vi "Calculate_(101)_Global_Cost_F()-1.vi"(5 "[IN] Still connect\ned tracks in group":T1, 6 "[IN] Max angle":dbl, 7 "[IN] Subtracks":T2(array[cluster]), 8 "error IN":errorcluster, 9 "[IN] Areas particles\nPrimary Detected":dbl[][](array[numeric]), 10 "[IN] Primary \n(X,Y) Detected":dbl[][](array[numeric]), 11 "[IN] Cost function":i8[](array[numeric])) -> (0 "error OUT":errorcluster, 3 "[OUT] Cost function":i8[](array[numeric]))   [LabVIEW 2013]
uses:
  <vilib>/Analysis/NI_AALBase.lvlib
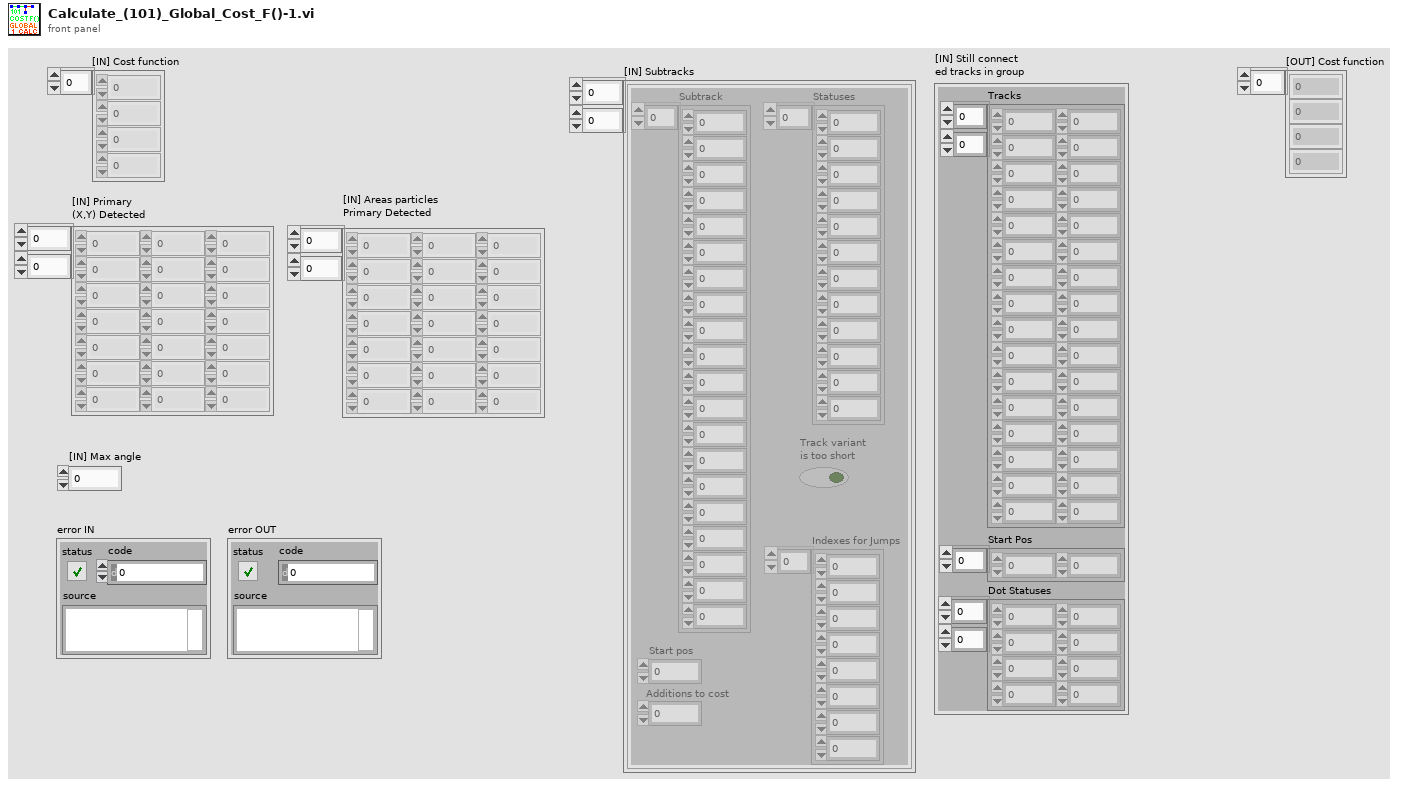
[diagram p1: front panel]
types:
  T1 = cluster{"Tracks":dbl[][], "Start Pos":i32[], "Dot Statuses":i16[][]}
  T2 = cluster{"Subtrack":dbl[], "Statuses":i16[], "Start pos":i32, "Additions to cost":i32, "Track variant \nis too short":bool, "Indexes for Jumps":i32[]}[][]
  T3 = cluster{"Subtrack":dbl[], "Statuses":i16[], "Start pos":i32, "Additions to cost":i32, "Track variant \nis too short":bool, "Indexes for Jumps":i32[]}[]
  T4 = cluster{"Subtrack":dbl[], "Statuses":i16[], "Start pos":i32, "Additions to cost":i32, "Track variant \nis too short":bool, "Indexes for Jumps":i32[]}
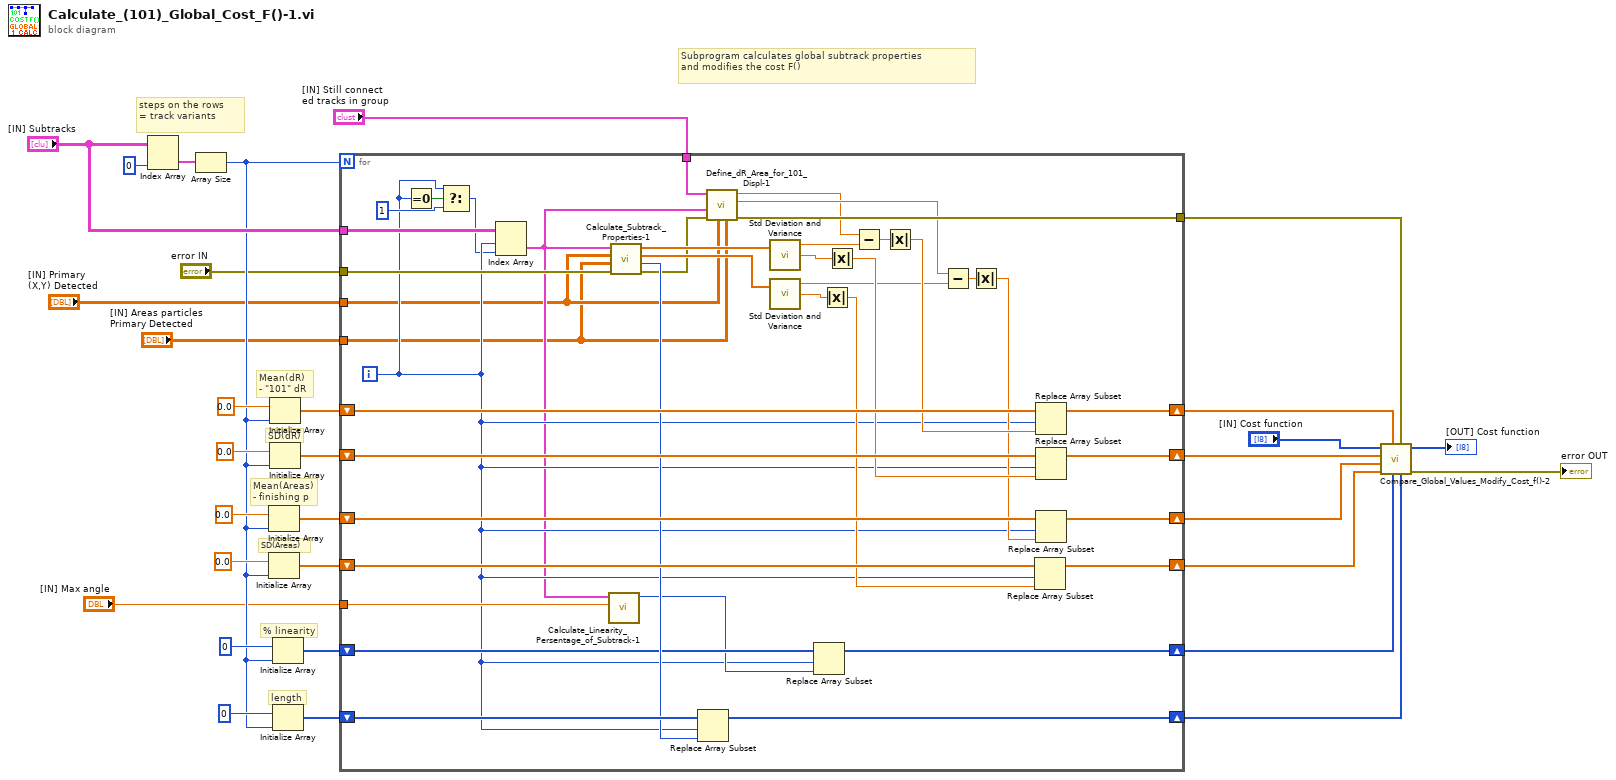
[diagram p0: block diagram]
diagram:
  # "Subprogram calculates global subtrack properties\nand modifies the cost F()"
  # "Mean(Areas)\n- finishing p"
  # "SD(Areas)"
  # "% linearity"
  # "length"
  # "Mean(dR)\n- \"101\" dR"
  # "SD(dR)"
  # "steps on the rows\n= track variants"
  n1 = Index Array(array="[IN] Subtracks", index (col)=0 ("disabled index (col)")) -> (element=w30:T3)  [unwired: 1 in]
  n2 = Array Size(array=w30) -> (size(s)=w20:i32)
  n3 = Initialize Array(0.0, w20) -> (w16:dbl[])
  n4 = Initialize Array(0.0, w20) -> (w15:dbl[])
  n5 = Initialize Array(0.0, w20) -> (w26:dbl[])
  n6 = Initialize Array(0.0, w20) -> (w25:dbl[])
  n7 = Initialize Array(u8 0, w20) -> (w11:u8[])
  n8 = Initialize Array(u8 0, w20) -> (w14:u8[])
  n9 = for {
    N: w20 -> [_]
    tunnel: "[IN] Subtracks" -> [w72]
    shift-right: [w66] -> w9
    shift-left: w26 -> [w69]
    shift-right: [w65] -> w7
    shift-left: w25 -> [w68]
    tunnel: "error IN" -> [w71]
    tunnel: "[IN] Primary \n(X,Y) Detected" -> [w35]
    tunnel: "[IN] Areas particles\nPrimary Detected" -> [w34]
    shift-right: [w59] -> w6
    shift-left: w16 -> [w64]
    shift-right: [w62] -> w5
    shift-left: w15 -> [w63]
    shift-right: [w54] -> w1
    shift-left: w14 -> [w56]
    tunnel: "[IN] Still connect\ned tracks in group" -> [w39]
    tunnel: "[IN] Max angle" -> [w47]
    shift-right: [w44] -> w2
    shift-left: w11 -> [w46]
    tunnel: [w36] -> w10
    i -> [w41]
    n10 = Equal To 0?(x=w41) -> (x = 0?=w43:bool)
    n11 = Select(t=w41, s=w43, f=1) -> (s? t:f=w40:i32)
    n12 = Index Array(array=w72, index (row)=w41, index (col)=w40) -> (element=w38:T4)
    n13 = call "Calculate_Linearity_Persentage_of_Subtrack-1.vi"("[IN] Max angle"=w47, "[IN] Subtrack"=w38) -> ("[OUT] Track Linearity in %"=w45:u8)  [unwired: 5 in]
    n14 = call "Calculate_Subtrack_Properties-1.vi"("error IN"=w71, "[IN] Areas particles\nPrimary Detected"=w34, "[IN] Primary \n(X,Y) Detected"=w35, "[IN] Subtrack"=w38) -> ("error OUT"=w37:errorcluster, "[OUT] Length of track"=w55:u8, "[OUT] Areas"=w67:dbl[], "[OUT] dR (displ)"=w70:dbl[])  [unwired: 2 in]
    n15 = Replace Array Subset(array=w56, new element=w55, index=w41) -> (w54:u8[])
    n16 = call "Define_dR_Area_for_101_Displ-1.vi"("[IN] Areas particles\nPrimary Detected"=w34, "[IN] Primary \n(X,Y) Detected"=w35, "error IN"=w37, "[IN] Subtrack"=w38, "[IN] Still connect\ned tracks in group"=w39) -> ("error OUT"=w36:errorcluster, "[OUT] Area of  \"101\" \ndestination point"=w33:dbl, "[OUT] dR for 101 \ndisplacement"=w32:dbl)  [unwired: 4 in]
    n17 = call <vilib>:"Std Deviation and Variance.vi"("X"=w70) -> ("mean"=w53:dbl, "standard deviation"=w61:dbl)  [unwired: 1 in, 1 out]
    n18 = call <vilib>:"Std Deviation and Variance.vi"("X"=w67) -> ("mean"=w50:dbl, "standard deviation"=w58:dbl)  [unwired: 1 in, 1 out]
    n19 = Replace Array Subset(array=w46, new element=w45, index=w41) -> (w44:u8[])
    n20 = Absolute Value(x=w58) -> (abs(x)=w57:dbl)
    n21 = Absolute Value(x=w61) -> (abs(x)=w60:dbl)
    n22 = Subtract(x=w32, y=w53) -> (x-y=w52:dbl)
    n23 = Absolute Value(x=w52) -> (abs(x)=w51:dbl)
    n24 = Subtract(x=w33, y=w50) -> (x-y=w49:dbl)
    n25 = Absolute Value(x=w49) -> (abs(x)=w48:dbl)
    n26 = Replace Array Subset(array=w63, new element=w57, index=w41) -> (w62:dbl[])
    n27 = Replace Array Subset(array=w69, new element=w51, index=w41) -> (w66:dbl[])
    n28 = Replace Array Subset(array=w68, new element=w60, index=w41) -> (w65:dbl[])
    n29 = Replace Array Subset(array=w64, new element=w48, index=w41) -> (w59:dbl[])
  }
  n30 = call "Compare_Global_Values_Modify_Cost_f()-2.vi"("[IN] Lengths"=w1, "error IN"=w10, "[IN] Linearity"=w2, "[IN] Array of Mean\n(dR) - Problem dR"=w9, "[IN] SD(Areas)"=w5, "[IN] Array of Mean(Areas)\n - Problem finish Area"=w6, "[IN] SD(dR)"=w7, "[IN] Cost function"="[IN] Cost function") -> ("error OUT"=→"error OUT":errorcluster, "[OUT] Cost function"=→"[OUT] Cost function":i8[])  [unwired: 2 in]
